vi "rad_Get Second Image Info.vi"(6 "Operation":T3, 7 "Comparison Image Path":path, 8 "error in (no error)":errorcluster, 9 "TempFolder Path":path, 10 "RT Target IP":string, 11 "Target settings in":T1={"Hostname"="", "Serial number"="", "Product name"="", "Product code"=0, "System status"="", "Credential type"=enum."None/Unlocked", "User added?"=FALSE, "Primary NIC"={"MAC address"="", "IP Address Request Mode"=2, "IP address"="", "Subnet mask"="", "Gateway"="", "DNS server"=""}} {"Primary NIC"."IP Address Request Mode" items=["Static"=1, "DHCP/Link-Local"=2, "Link-Local Only"=4, "DHCP Only"=8]}) -> (0 "error out":errorcluster, 1 "AppImage Properties":T4, 2 "Unzipped App Image Folder Path":path, 3 "Target settings out":T1={"Hostname"="", "Serial number"="", "Product name"="", "Product code"=0, "System status"="", "Credential type"=enum."None/Unlocked", "User added?"=FALSE, "Primary NIC"={"MAC address"="", "IP Address Request Mode"=2, "IP address"="", "Subnet mask"="", "Gateway"="", "DNS server"=""}} {"Primary NIC"."IP Address Request Mode" items=["Static"=1, "DHCP/Link-Local"=2, "Link-Local Only"=4, "DHCP Only"=8]})   [LabVIEW 2014]
uses:
  App Images/TypeDefs/rad_FPGA Flash Properties.ctl
  App Images/TypeDefs/rad_FPGA Properties.ctl
  App Images/TypeDefs/rad_Application Image Properties.ctl
  TypeDefs/rad_Comparison Modes.ctl
  Targets/TypeDefs/rad_Target Information.ctl
  Targets/TypeDefs/rad_Target Network Settings.ctl
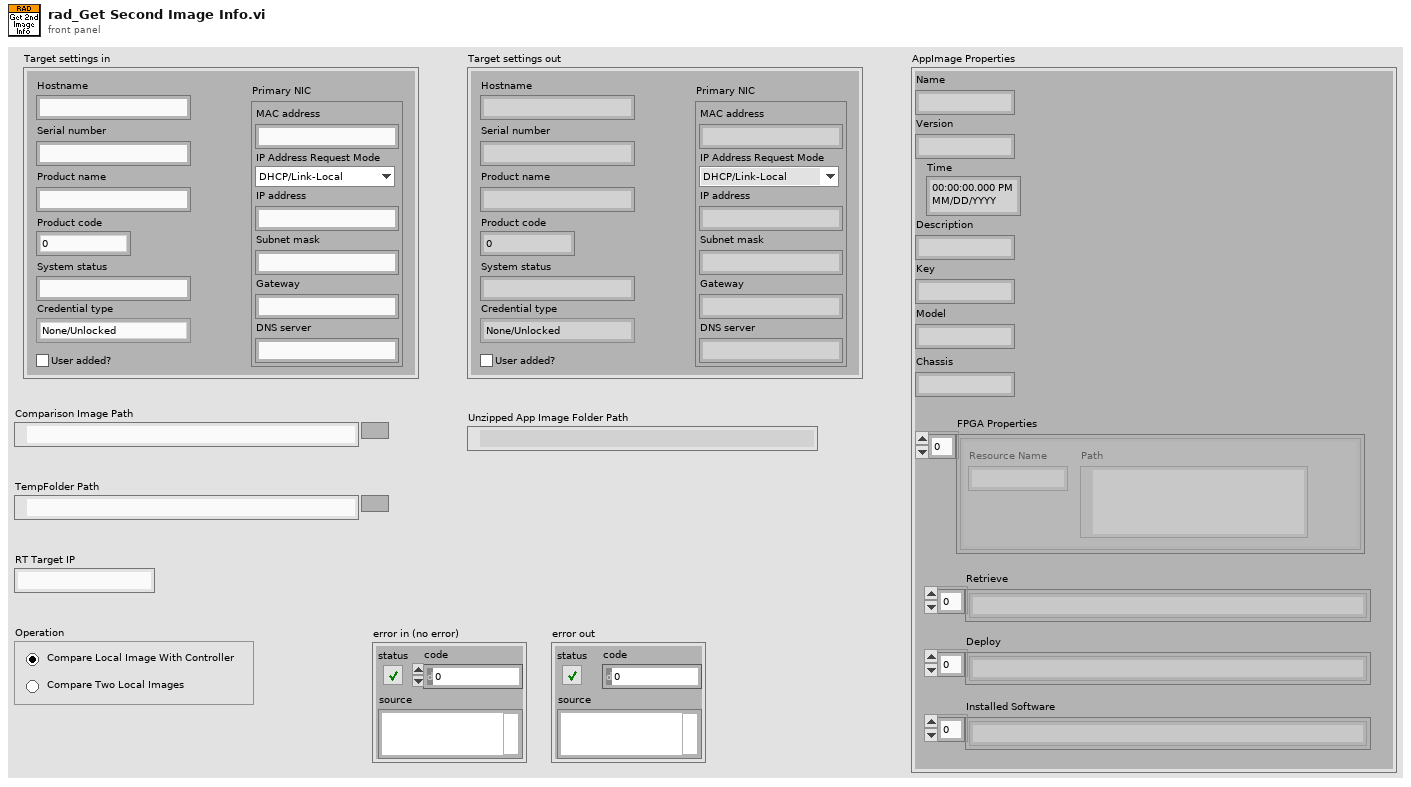
[diagram p1: front panel]
types:
  T1 = typedef "rad_Target Information.ctl" = cluster{"Hostname":string, "Serial number":string, "Product name":string, "Product code":i32, "System status":string, "Credential type":enum16{"None/Unlocked", "FTP Password", "NIAuth Credentials"}, "User added?":bool, "Primary NIC":T2}
  T2 = typedef "rad_Target Network Settings.ctl" = cluster{"MAC address":string, "IP Address Request Mode":i32, "IP address":string, "Subnet mask":string, "Gateway":string, "DNS server":string}
  T3 = typedef "rad_Comparison Modes.ctl" = enum32{"Compare Local Image With Controller", "Compare Two Local Images"}
  T4 = typedef "rad_Application Image Properties.ctl" = cluster{"Name":string, "Version":string, "Time":timestamp, "Description":string, "Key":string, "Chassis":string, "FPGA Properties":T5, "Model":string, "Retrieve":string[], "Deploy":string[], "Installed Software":string[]}
  T5 = typedef "rad_FPGA Properties.ctl" = T6[]
  T6 = typedef "rad_FPGA Flash Properties.ctl" = cluster{"Resource Name":string, "Path":path}
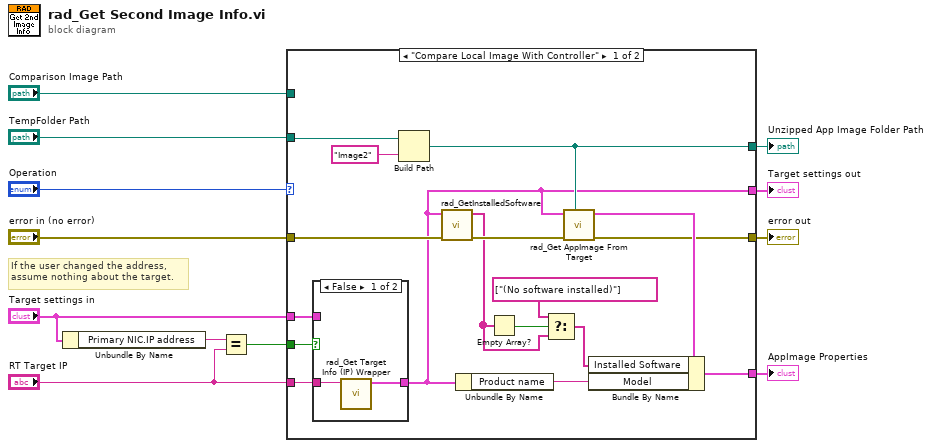
[diagram p0: block diagram]
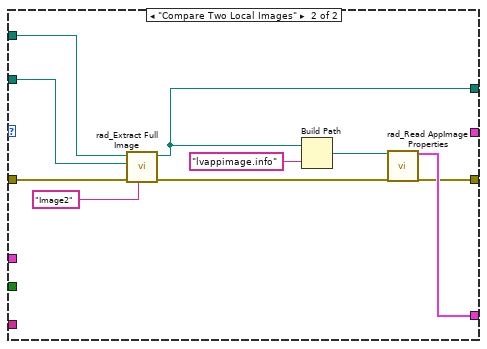
[diagram p3: hidden frame]
diagram:
  # "If the user changed the address,\nassume nothing about the target."
  n1 = Unbundle By Name("Target settings in") -> ("Primary NIC.IP address"=w5:string)
  n2 = Equal?(x=w5, y="RT Target IP") -> (x = y?=w6:bool)
  n3 = case shown="\"Compare Local Image With Controller\"" "Operation" {
    tunnel: [w18 w34] -> w11
    tunnel: "error in (no error)" -> [w20 w40]
    tunnel: [w24 w37] -> w2
    tunnel: "TempFolder Path" -> [w28 w42]
    tunnel: "Target settings in" -> [w26 _]
    tunnel: w6 -> [w27 _]
    tunnel: "RT Target IP" -> [w25 _]
    tunnel: [w23 w35] -> w10
    tunnel: "Comparison Image Path" -> [_ w33]
    tunnel: [w17 _] -> w1
    frame "Compare Local Image With Controller" {
      n4 = case shown="False" w27 {
        tunnel: w26 -> [_ w32]
        tunnel: [w30 w32] -> w17
        tunnel: w25 -> [w31 _]
        frame False {
          n5 = call "rad_Get Target Info (IP) Wrapper.vi"("target address"=w31) -> ("Target settings"=w30:T1)  [unwired: 9 in, 1 out]
        }
        frame True {
        }
      }
      n6 = Build Path(base path=w28, name or relative path="Image2") -> (appended path=w24:path)
      n7 = call "rad_GetInstalledSoftware.vi"("error in (no error)"=w20, "Target settings"=w17) -> ("error out"=w19:errorcluster, "installedSoftware"=w15:string[])  [unwired: 8 in]
      n8 = Unbundle By Name(w17) -> ("Product name"=w22:string)
      n9 = Empty Array?(array=w15) -> (empty?=w16:bool)
      n10 = Select(t=string[] ["(No software installed)"], s=w16, f=w15) -> (s? t:f=w14:string[])
      n11 = call "rad_Get AppImage From Target.vi"("Temp Folder"=w24, "error in (no error)"=w19, "Target settings"=w17) -> ("error out"=w18:errorcluster, "AppImage Properties"=w21:T4)  [unwired: 6 in, 1 out]
      n12 = Bundle By Name(cluster=w21, "Installed Software"=w14, "Model"=w22) -> (w23:T4)
    }
    frame "Compare Two Local Images" {
      n13 = call "rad_Extract Full Image.vi"("Subfolder (lvappimage.contents)"="Image2" ("name or relative path"), "error in (no error)"=w40, "App Image Temp Folder"=w42, "Zipped App Image File Path"=w33) -> ("error out"=w36:errorcluster, "Unzipped App Image Folder Path"=w37:path)  [unwired: 6 in]
      n14 = Build Path(base path=w37, name or relative path="lvappimage.info") -> (appended path=w39:path)
      n15 = call "rad_Read AppImage Properties.vi"("AppImage Properties Path"=w39, "error in (no error)"=w36) -> ("AppImage Properties"=w35:T4, "error out"=w34:errorcluster)  [unwired: 12 in, 4 out]
    }
  }
  "error out" <- w11
  "AppImage Properties" <- w10
  "Unzipped App Image Folder Path" <- w2
  "Target settings out" <- w1
